vi "数值变字符串输出.vi"(1 "浮点数值":dbl, 2 "小数点":dbl) -> (0 "输出字符串":string)   [LabVIEW 2016]
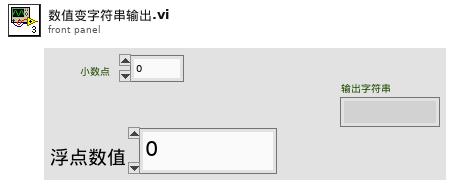
[diagram p1: front panel]
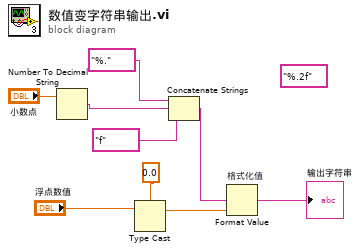
[diagram p0: block diagram]
diagram:
  (unwired) "%.2f" ("格式字符串")
  n1 = Number To Decimal String(number="小数点") -> (decimal integer string=w2:string)  [unwired: 1 in]
  n2 = Type Cast(type=0.0 ("类型"), x="浮点数值") -> (*(type *) &x=w7:dbl)
  n3 = Concatenate Strings("%." ("格式字符串"), w2, "f" ("格式字符串")) -> (w5:string)
  n4 = Format Value "格式化值"(format string=w5, value (0)=w7) -> (output string=→"输出字符串":string)  [unwired: 1 in]
